vi "set_autostart_flag.vi"(8 "error in (no error)":errorcluster, 10 "autostart?":bool, 11 "GenericScanMode in":refnum<class "GenericImagingMode.lvclass">) -> (0 "error out":errorcluster, 3 "GenericScanMode out":refnum<class "GenericImagingMode.lvclass">)   [LabVIEW 2010, in "GenericImagingMode.lvclass"]
uses:
  GenericImagingMode.lvclass
  GenericImagingMode.lvclass/GenericImagingMode.ctl
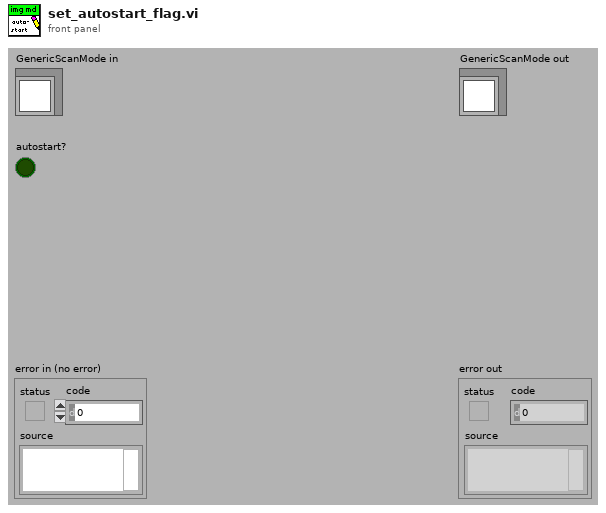
[diagram p1: front panel]
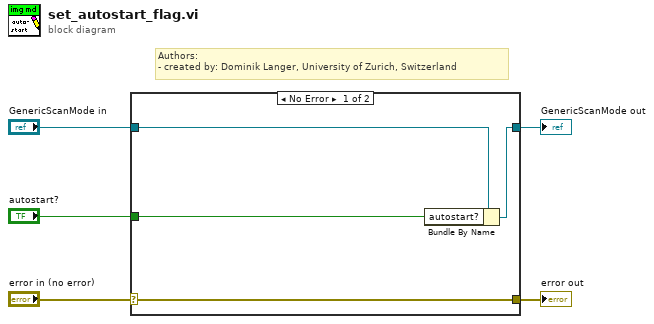
[diagram p0: block diagram]
diagram:
  # "Authors: \n- created by: Dominik Langer, University of Zurich, Switzerland"
  n1 = case shown="No Error" "error in (no error)" {
    selector: "error in (no error)" -> [w9 w10]
    tunnel: [w9 w10] -> w4
    tunnel: [w7 w11] -> w2
    tunnel: "GenericScanMode in" -> [w8 w11]
    tunnel: "autostart?" -> [w6 _]
    frame No Error {
      n2 = Bundle By Name(cluster=w8, "autostart?"=w6) -> (w7:refnum<class "GenericImagingMode.lvclass">)
    }
    frame Error {
    }
  }
  "error out" <- w4
  "GenericScanMode out" <- w2
